vi "Unregister GUI.vi"(8 "error in (no error)":errorcluster, 11 "GUI Helper in":refnum<class "GUI Helper.lvclass">) -> (0 "error out":errorcluster, 3 "GUI Helper out":refnum<class "GUI Helper.lvclass">)   [LabVIEW 2020, in "VolatusGUI.lvlib" / "GUI Helper.lvclass"]
uses:
  GUI Helper.lvclass
  Unregister GUI.ctl
  GUI Helper.lvclass/GUI Helper.ctl
  Volatus/MessageQ/MessageQ.lvclass/MessageQ.ctl
  Volatus/MessageQ/MessageQ.lvclass
  VolatusGUI.lvlib
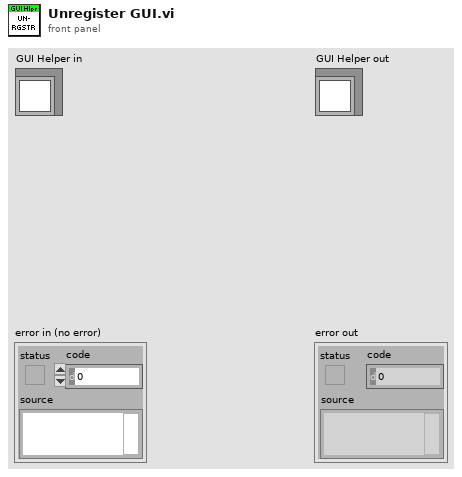
[diagram p1: front panel]
types:
  T1 = typedef "VolatusGUI.lvlib/Unregister GUI.ctl" = cluster{"Name":string}
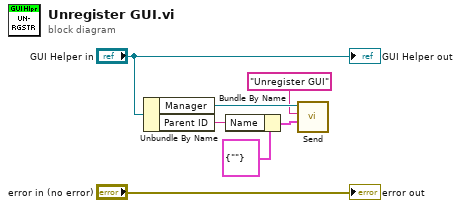
[diagram p0: block diagram]
diagram:
  n1 = Unbundle By Name("GUI Helper in") -> ("Manager"=w5:refnum<class "MessageQ.lvclass">, "Parent ID"=w2:string)
  n2 = Bundle By Name(cluster=T1 {"Name"=""} ("Unregister GUI"), "Name"=w2) -> (w1:T1)
  n3 = call "Send.vi"("Data"=w1, "ID"="Unregister GUI", "MessageQ in"=w5) -> ()  [unwired: 7 in, 2 out]
  "error out" <- "error in (no error)"
  "GUI Helper out" <- "GUI Helper in"
